vi "Hardware Config.vi"() -> ()   [LabVIEW 2022 SP3]
uses:
  Controls/Config.ctl
  Global 1.vi
panel:
  in  "Signal list":bool
  out "Config":T1={"AO config"=[], "AI config"=[], "DI config"=[], "DO config"=[], "TC config"=[{"Channel_Name"="", "Channel_Number"="", "Pre_Scale_min"=0.0, "Pre_Scale_max"=0.0, "units"=4, " type"=7}], "ACC config"=[], "SG config"=[], "Strain Gauge Settings"={"poisson ratio"=0.3, "nominal gage resistance"=120.0, "gage factor"=2.08}, "bridge information"={"strain configuration"=10271, "lead wire resistance"=1.7, "initial bridge voltage"=0.0, "voltage excitation source"=10200, "voltage excitation value"=3.3}, "Sample Rate"={"AI Sample Rate"=0.0, "AO Sample Rate"=0.0, "DI Sample Rate"=0.0, "TC Sample Rate"=0.0, "DO Sample Rate"=0.0, "SG Sample Rate"=0.0, "ACC Sample Rate"=0.0}} {"bridge information"."voltage excitation source" items=["Internal"=10200, "External"=10167, "None"=10230]; "bridge information"."voltage excitation value" format="%0.2f"; "bridge information"."lead wire resistance" format="%0.2f"; "bridge information"."strain configuration" items=["Full Bridge I"=10183, "Full Bridge II"=10184, "Full Bridge III"=10185, "Half Bridge I"=10188, "Half Bridge II"=10189, "Quarter Bridge I"=10271, "Quarter Bridge II"=10272]; "ACC config"."Terminal configuration" items=["default"=-1, "RSE"=10083, "NRSE"=10078, "Differential"=10106, "Pseudodifferential"=12529]; "ACC config"."Sensitivity units" items=["mVolts/g"=12509, "Volts/g"=12510]; "TC config"."type" items=["J"=10072, "K"=10073, "N"=10077, "R"=10082, "S"=10085, "T"=10086, "B"=10047, "E"=10055]; "TC config"."units" items=["Deg C", "Deg F", "Kelvins", "Deg R", "From Custom Scale"]}
  in  "Cancel":bool
  in  "Load Configuration":bool
  in  "New configuration":bool
  in  "Save Config":bool
  in  "Tab Control":T2(tab)
  in  "DO Sample Rate":dbl format="%#_g Hz"
  in  "DO config":T3(array[cluster])=[{"Channel_Name"="", "Channel_Number"="", "Default_Value"=FALSE, "Units"=FALSE}]
  in  "DI Sample Rate":dbl format="%#_g Hz"
  in  "DI config":T3(array[cluster])
  in  "AO Sample Rate":dbl format="%#_g Hz"
  in  "AO config":T4(array[cluster])
  in  "AI Sample Rate":dbl format="%#_g Hz"
  in  "AI config":T5(array[cluster])
  in  "TC Sample Rate":dbl format="%#_g Hz"
  in  "TC config":T6(array[cluster]) {"thermocouple type" items=["J", "K", "N", "R", "S", "T", "B", "E"]; "units" items=["Deg C", "Deg F", "Kelvins", "Deg R", "From Custom Scale"]}
  in  "ACC Sample Rate":dbl format="%#_g Hz"
  in  "ACC config":T7(array[cluster]) {"Sensitivity units" items=["mVolts/g"=12509, "Volts/g"=12510]; "Terminal configuration" items=["default"=-1, "RSE"=10083, "NRSE"=10078, "Differential"=10106, "Pseudodifferential"=12529]}
  in  "SG Sample Rate":dbl format="%#_g Hz"
  in  "SG config":T8(array[cluster])
  in  "SG Settings":T9={"gage factor"=2.08, "nominal gage \nresistance"=120.0, "poisson ratio"=0.3}
  in  "Bridge Settings":T10={"strain configuration"=10271, "lead wire resistance"=1.7, "initial bridge voltage"=0.0, "voltage excitation source"=10200, "voltage excitation value"=3.3} {"strain configuration" items=["Full Bridge I"=10183, "Full Bridge II"=10184, "Full Bridge III"=10185, "Half Bridge I"=10188, "Half Bridge II"=10189, "Quarter Bridge I"=10271, "Quarter Bridge II"=10272]; "voltage excitation source" items=["Internal"=10200, "External"=10167, "None"=10230]}
  # "DO_Channel_Name"
  # "DO_Channel_Number"
  # "Default Value"
  # "Invert?"
  # "DI_Channel_Name"
  # "DI_Channel_Number"
  # "Default Value"
  # "Invert?"
  # "AO_Channel_Name"
  # "AO_Channel_Number"
  # "Default Value"
  # "Units"
  # "AI_Channel_Name"
  # "AI_Channel_Number"
  # "Pre_Scale_min"
  # "Pre_Scale_max"
  # "Scale_min"
  # "Scale_max"
  # "Units"
  # "TC_Channel_Name"
  # "TC_Channel_Number"
  # "Max_Value"
  # "Units"
  # "Type"
  # "Min_Value"
  # "ACC_Channel_Name"
  # "ACC_Channel_Number"
  # "Min_Value"
  # "Max_Value"
  # "Terminal Config"
  # "Sensitivity"
  # "Sensitivity Units"
  # "SG_Channel_Name"
  # "SG_Channel_Number"
  # "Min_Value"
  # "Max_Value"
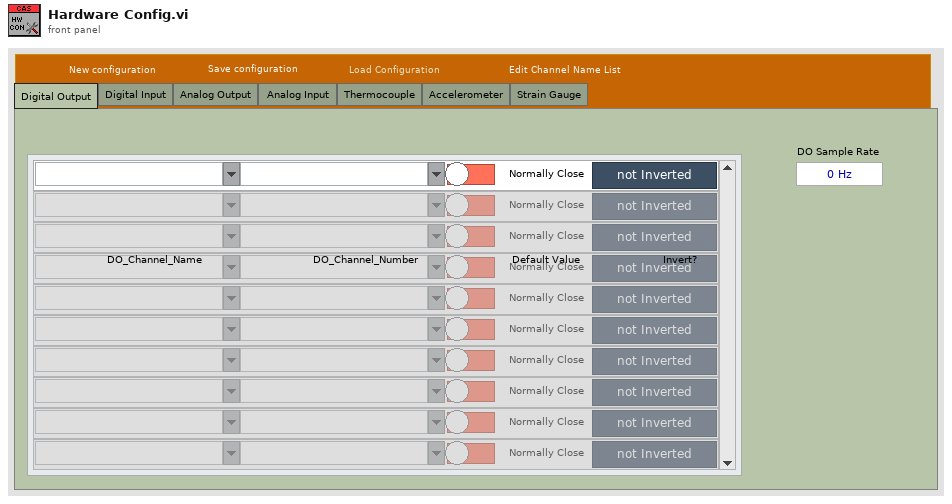
[diagram p1: front panel]
types:
  T1 = typedef "Config.ctl" = cluster{"AO config":cluster{"Channel_Name":string, "Channel_Number":string, "Default_Value":dbl, "Units":string}[], "AI config":cluster{"Channel_Name":string, "Channel_Number":string, "Pre_Scale_min":dbl, "Pre_Scale_max":dbl, "Sensor_min":dbl, "Sensor_max":dbl, "Units":string}[], "DI config":cluster{"Channel_Name":string, "Channel_Number":string, "Default_Value":bool, "DI invert?":bool}[], "DO config":cluster{"Channel_Name":string, "Channel_Number":string, "Default_Value":bool, "DO invert?":bool}[], "TC config":cluster{"Channel_Name":string, "Channel_Number":string, "Pre_Scale_min":dbl, "Pre_Scale_max":dbl, "units":i32, " type":i32}[], "ACC config":cluster{"Channel_Name":string, "Channel_Number":string, "Pre_Scale_min":dbl, "Pre_Scale_max":dbl, "Terminal configuration":i32, "Sensitivity":dbl, "Sensitivity units":i32}[], "SG config":cluster{"Channel_Name":string, "Channel_Number":string, "Pre_Scale_min":dbl, "Pre_Scale_max":dbl}[], "Strain Gauge Settings":cluster{"poisson ratio":dbl, "nominal gage resistance":dbl, "gage factor":dbl}, "bridge information":cluster{"strain configuration":i32, "lead wire resistance":dbl, "initial bridge voltage":dbl, "voltage excitation source":i32, "voltage excitation value":dbl}, "Sample Rate":cluster{"AI Sample Rate":dbl, "AO Sample Rate":dbl, "DI Sample Rate":dbl, "TC Sample Rate":dbl, "DO Sample Rate":dbl, "SG Sample Rate":dbl, "ACC Sample Rate":dbl}}
  T2 = enum32{"Digital Output", "Digital Input", "Analog Output", "Analog Input ", "Thermocouple", "Accelerometer", "Strain Gauge"}
  T3 = cluster{"Channel_Name":string, "Channel_Number":string, "Default_Value":bool, "Units":bool}[]
  T4 = cluster{"Channel_Name":string, "Channel_Number":string, "Default_Value":dbl, "Units":string}[]
  T5 = cluster{"Channel_Name":string, "Channel_Number":string, "Pre_Scale_min":dbl, "Pre_Scale_max":dbl, "Sensor_min":dbl, "Sensor_max":dbl, "Units":string}[]
  T6 = cluster{"Channel_Name":string, "Channel_Number":string, "Pre_Scale_min":dbl, "Pre_Scale_max":dbl, "units":i32, "thermocouple type":i32}[]
  T7 = cluster{"Channel_Name":string, "Channel_Number":string, "Pre_Scale_min":dbl, "Pre_Scale_max":dbl, "Terminal configuration":i32, "Sensitivity":dbl, "Sensitivity units":i32}[]
  T8 = cluster{"Channel_Name":string, "Channel_Number":string, "Pre_Scale_min":dbl, "Pre_Scale_max":dbl}[]
  T9 = cluster{"gage factor":dbl, "nominal gage \nresistance":dbl, "poisson ratio":dbl}
  T10 = cluster{"strain configuration":i32, "lead wire resistance":dbl, "initial bridge voltage":dbl, "voltage excitation source":i32, "voltage excitation value":dbl}
  T11 = cluster{"Data":T1, "path":path, "Name ref":refnum<vi>[], "Names":string[][], "Signal path":path, "SR":cluster{"AI Sample Rate":dbl, "AO Sample Rate":dbl, "DI Sample Rate":dbl, "TC Sample Rate":dbl, "DO Sample Rate":dbl, "SG Sample Rate":dbl, "ACC Sample Rate":dbl}}
  T12 = typedef "Root path.ctl" = cluster{"Data":path, "Sub VI's":path, "Source code":path}
  T13 = cluster{"AI":string[], "DI":string[], "DO":string[], "SG":string[], "AO":string[], "TC":string[], "ACC":string[]}
  T14 = cluster{"AI Channel list":tag[], "AO Channel list":tag[], "DO Channel list ":tag[], "DI Channel list":tag[]}
  T15 = cluster{"AI Sample Rate":dbl, "AO Sample Rate":dbl, "DI Sample Rate":dbl, "TC Sample Rate":dbl, "DO Sample Rate":dbl, "SG Sample Rate":dbl, "ACC Sample Rate":dbl}
  T16 = enum16{"open", "replace", "create", "open or create", "replace or create", "replace or create with confirmation"}
  T17 = enum32{"Invalid", "Standard", "Closed", "Hidden", "Minimized", "Maximized"}
  T18 = cluster{"Channel_Name":string, "Channel_Number":string, "Default_Value":bool, "DI invert?":bool}[]
  T19 = cluster{"Channel_Name":string, "Channel_Number":string, "Default_Value":bool, "DO invert?":bool}[]
  T20 = cluster{"Channel_Name":string, "Channel_Number":string, "Pre_Scale_min":dbl, "Pre_Scale_max":dbl, "units":i32, " type":i32}[]
  T21 = cluster{"poisson ratio":dbl, "nominal gage resistance":dbl, "gage factor":dbl}
  T22 = cluster{"Channel_Name":string, "Channel_Number":string}
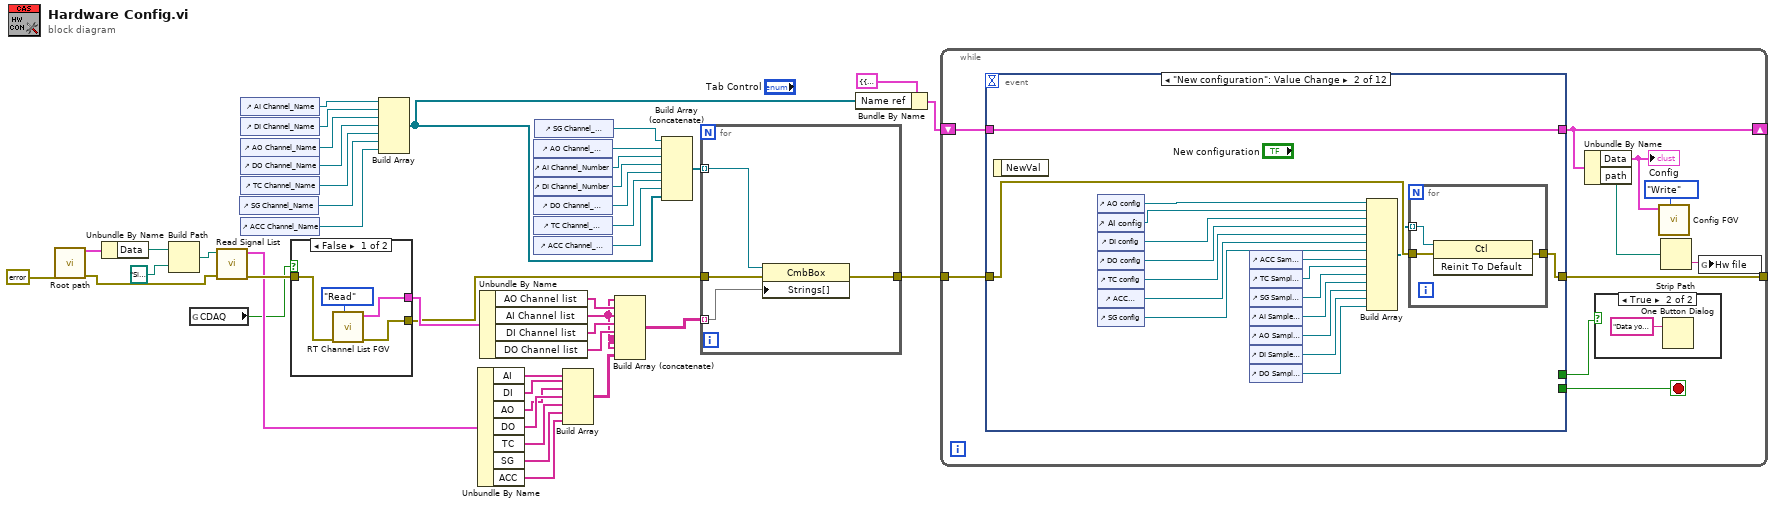
[diagram p0: block diagram]
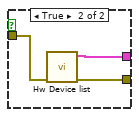
[diagram p2: hidden frame]
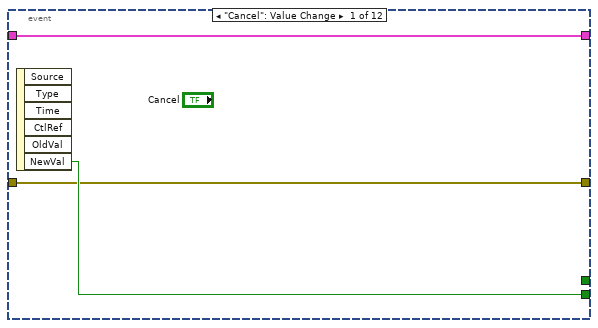
[diagram p4: hidden frame]
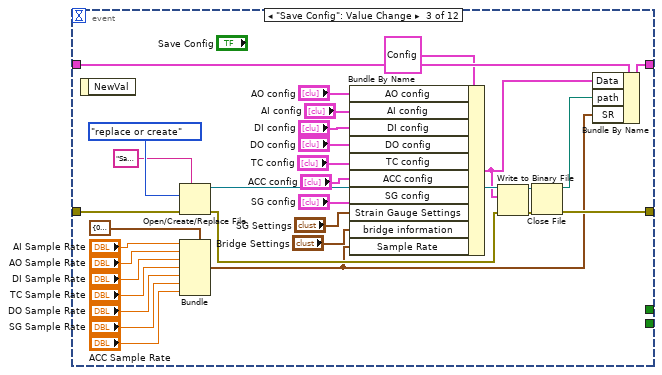
[diagram p5: hidden frame]
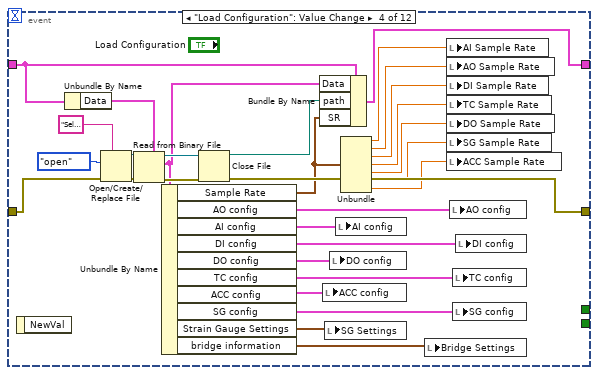
[diagram p6: hidden frame]
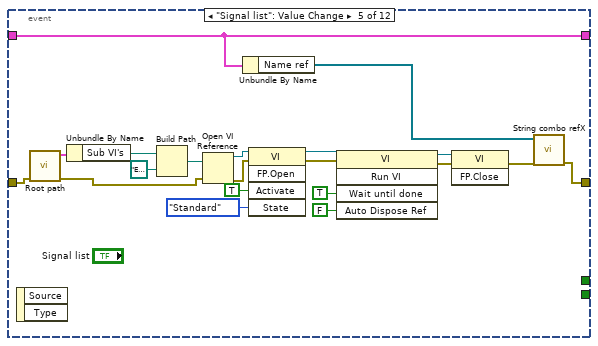
[diagram p7: hidden frame]
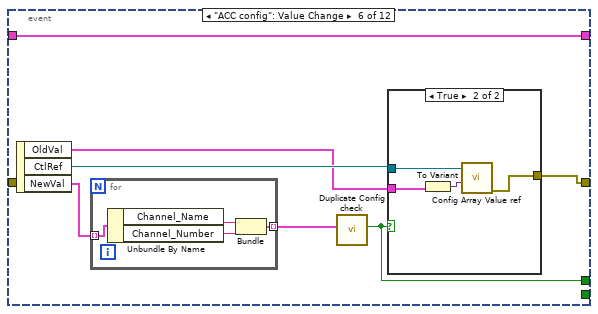
[diagram p8: hidden frame]
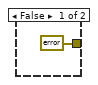
[diagram p9: hidden frame]
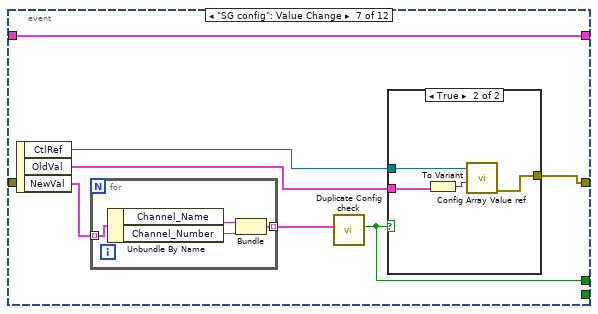
[diagram p10: hidden frame]
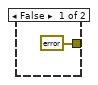
[diagram p11: hidden frame]
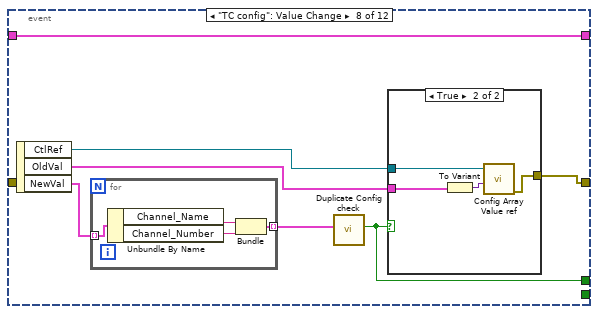
[diagram p12: hidden frame]
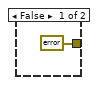
[diagram p13: hidden frame]
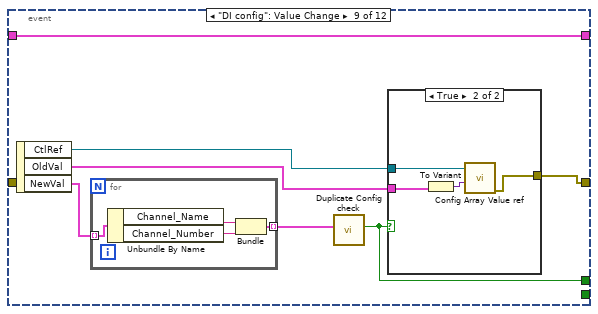
[diagram p14: hidden frame]
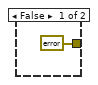
[diagram p15: hidden frame]
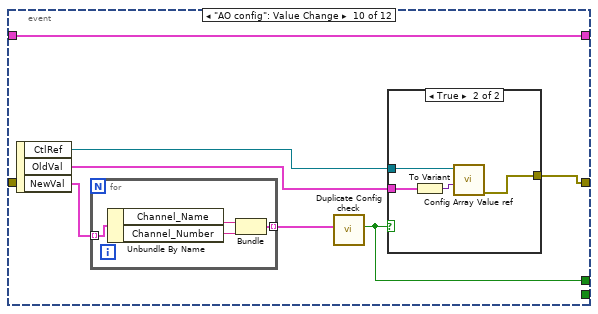
[diagram p16: hidden frame]
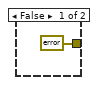
[diagram p17: hidden frame]
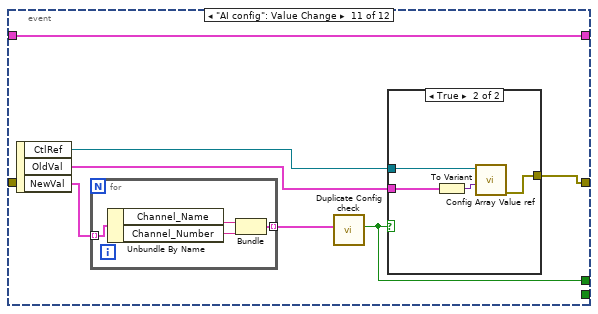
[diagram p18: hidden frame]
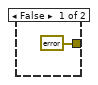
[diagram p19: hidden frame]
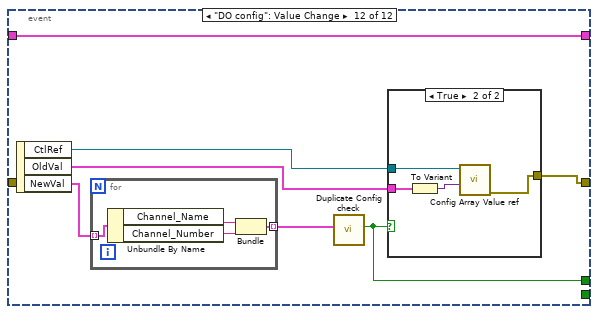
[diagram p20: hidden frame]
diagram:
  n1 = call "Root path.vi"("error in (no error)"=errorcluster {"status"=FALSE, "code"=0, "source"=""} ("error in")) -> ("error out"=w18:errorcluster, "Root Path"=w25:T12)  [unwired: 9 in]
  n2 = Unbundle By Name(w25) -> ("Data"=w24:path)
  n3 = Build Path(base path=w24, name or relative path=path "Signal list/Signal1") -> (appended path=w22:path)
  n4 = global read "Global 1.vi" "CDAQ"() -> (w1:bool)
  n5 = call "Read Signal List.vi"("error in"=w18, "file path (use dialog)"=w22) -> ("error out"=w27:errorcluster, "Names"=w17:T13)  [unwired: 8 in]
  n6 = control-ref of="SG Channel_Name"() -> (w3:refnum<vi>)
  n7 = control-ref of="AI Channel_Name"() -> (w21:refnum<vi>)
  n8 = control-ref of="DI Channel_Name"() -> (w20:refnum<vi>)
  n9 = control-ref of="AO Channel_Name"() -> (w5:refnum<vi>)
  n10 = control-ref of="DO Channel_Name"() -> (w4:refnum<vi>)
  n11 = control-ref of="TC Channel_Name"() -> (w19:refnum<vi>)
  n12 = control-ref of="ACC Channel_Name"() -> (w2:refnum<vi>)
  n13 = case shown="False" w1 {
    tunnel: [w46 w50] -> w35
    tunnel: [w45 w49] -> w34
    tunnel: w27 -> [w44 w48]
    frame False {
      n14 = call "RT Channel List FGV.vi"("Enum"=enum16{"Read", "Write"}."Read", "error in (no error)"=w44) -> ("error out"=w45:errorcluster, "Channel List"=w46:T14)  [unwired: 8 in]
    }
    frame True {
      n15 = call "Hw Device list.vi"("error in (no error)"=w48) -> ("error out"=w49:errorcluster, "Channel List"=w50:T14)  [unwired: 9 in]
    }
  }
  n16 = Build Array(w21, w20, w5, w4, w19, w3, w2) -> (w6:refnum<vi>[])
  n17 = Unbundle By Name(w17) -> ("AI"=w16:string[], "DI"=w15:string[], "AO"=w10:string[], "DO"=w14:string[], "TC"=w13:string[], "SG"=w12:string[], "ACC"=w11:string[])
  n18 = Unbundle By Name(w35) -> ("AO Channel list"=w29:tag[], "AI Channel list"=w28:tag[], "DI Channel list"=w38:tag[], "DO Channel list"=w37:tag[])
  n19 = control-ref of="AO Channel_Number"() -> (w43:refnum<vi>)
  n20 = control-ref of="AI Channel_Number"() -> (w42:refnum<vi>)
  n21 = control-ref of="DI Channel_Number"() -> (w41:refnum<vi>)
  n22 = control-ref of="DO Channel_Number"() -> (w40:refnum<vi>)
  n23 = control-ref of="TC Channel_Number"() -> (w32:refnum<vi>)
  n24 = control-ref of="ACC Channel_Number"() -> (w31:refnum<vi>)
  n25 = control-ref of="SG Channel_Number"() -> (w30:refnum<vi>)
  n26 = Build Array(w16, w15, w10, w14, w13, w12, w11) -> (w9:string[][])
  n27 = Build Array (concatenate)(w28, w29, w28, w38, w37, w28, w28, w9) -> (w36:string[][])
  n28 = Build Array (concatenate)(w30, w43, w42, w41, w40, w32, w31, w6) -> (w39:refnum<vi>[])
  n29 = for {
    tunnel: w39 -> [w54] mode=indexing
    tunnel: w36 -> [w51] mode=indexing
    tunnel: [w53] -> w33
    tunnel: w34 -> [w52]
    n30 = property class="CmbBox"(reference=w54, error in=w52, "Strings[]"=w51) -> (error out=w53:errorcluster)  [unwired: 1 out]
  }
  n31 = Bundle By Name(cluster=T11 {"Data"={"AO config"=[], "AI config"=[], "DI config"=[], "DO config"=[], "TC config"=[{"Channel_Name"="", "Channel_Number"="", "Pre_Scale_min"=0.0, "Pre_Scale_max"=0.0, "units"=4, " type"=7}], "ACC config"=[], "SG config"=[], "Strain Gauge Settings"={"poisson ratio"=0.3, "nominal gage resistance"=120.0, "gage factor"=2.08}, "bridge information"={"strain configuration"=10271, "lead wire resistance"=1.7, "initial bridge voltage"=0.0, "voltage excitation source"=10200, "voltage excitation value"=3.3}, "Sample Rate"={"AI Sample Rate"=0.0, "AO Sample Rate"=0.0, "DI Sample Rate"=0.0, "TC Sample Rate"=0.0, "DO Sample Rate"=0.0, "SG Sample Rate"=0.0, "ACC Sample Rate"=0.0}}, "path"=path "", "Name ref"=[], "Names"=[], "Signal path"=path "", "SR"={"AI Sample Rate"=0.0, "AO Sample Rate"=0.0, "DI Sample Rate"=0.0, "TC Sample Rate"=0.0, "DO Sample Rate"=0.0, "SG Sample Rate"=0.0, "ACC Sample Rate"=0.0}}, "Name ref"=w6) -> (w8:T11)
  n32 = while {
    shift-right: [w60] -> _
    shift-left: w8 -> [w61]
    tunnel: w33 -> [w63]
    tunnel: [w62] -> _
    stop <- w64 stop-if-true
    n33 = event shown="[1] \"New configuration\": Value Change" {
      selector: _ -> [_ _ _ _ _ _ _ _ _ _ _ _]
      dyn-events: _ -> [_ _ _ _ _ _ _ _ _ _ _ _]
      timeout: _ -> [_ _ _ _ _ _ _ _ _ _ _ _]
      tunnel: [w67 _ _ _ _ _ _ _ _ _ _ _] -> w64
      tunnel: w63 -> [w66 w86 w120 w150 w170 _ _ _ _ _ _ _]
      tunnel: [w66 w85 w115 w146 w151 w172 w190 w206 w222 w238 w254 w270] -> w62
      tunnel: w61 -> [w68 w84 w118 w140 w154 w177 w193 w209 w225 w241 w257 w273]
      tunnel: [w68 w84 w107 w141 w154 w177 w193 w209 w225 w241 w257 w273] -> w60
      tunnel: [_ _ _ _ _ w171 w187 w203 w219 w235 w251 w267] -> w55
      event "Cancel": Value Change {
        n34 = event-data() -> ("NewVal"=w67:bool)  [unwired: 1 in, 5 out]
      }
      event "New configuration": Value Change {
        n35 = event-data() -> ()  [unwired: 1 in, 1 out]
        n36 = control-ref of="AO config"() -> (w79:refnum<vi>)
        n37 = control-ref of="AI config"() -> (w80:refnum<vi>)
        n38 = control-ref of="DI config"() -> (w81:refnum<vi>)
        n39 = control-ref of="DO config"() -> (w82:refnum<vi>)
        n40 = control-ref of="TC config"() -> (w78:refnum<vi>)
        n41 = control-ref of="ACC config"() -> (w77:refnum<vi>)
        n42 = control-ref of="SG config"() -> (w76:refnum<vi>)
        n43 = control-ref of="ACC Sample Rate"() -> (w75:refnum<vi>)
        n44 = control-ref of="TC Sample Rate"() -> (w74:refnum<vi>)
        n45 = control-ref of="SG Sample Rate"() -> (w73:refnum<vi>)
        n46 = control-ref of="AI Sample Rate"() -> (w72:refnum<vi>)
        n47 = control-ref of="AO Sample Rate"() -> (w71:refnum<vi>)
        n48 = control-ref of="DI Sample Rate"() -> (w70:refnum<vi>)
        n49 = control-ref of="DO Sample Rate"() -> (w69:refnum<vi>)
        n50 = Build Array(w79, w80, w81, w82, w78, w77, w76, w75, w74, w73, w72, w71, w70, w69) -> (w83:refnum<vi>[])
        n51 = for {
          tunnel: w83 -> [w89] mode=indexing
          tunnel: w86 -> [w88]
          tunnel: [w87] -> w85
          n52 = invoke class="Ctl" method="Reinit To Default"(reference=w89, error in=w88) -> (error out=w87:errorcluster)  [unwired: 1 in, 2 out]
        }
      }
      event "Save Config": Value Change {
        n53 = event-data() -> ()  [unwired: 1 in, 1 out]
        n54 = Open/Create/Replace File(error in=w120, prompt="Save Changes", operation (0:open)=T16."replace or create") -> (refnum out=w114:refnum<file>, error out=w119:errorcluster)  [unwired: 3 in, 1 out]
        n55 = Bundle(cluster=T15 {"AI Sample Rate"=0.0, "AO Sample Rate"=0.0, "DI Sample Rate"=0.0, "TC Sample Rate"=0.0, "DO Sample Rate"=0.0, "SG Sample Rate"=0.0, "ACC Sample Rate"=0.0} ("Sample Rate"), "AI Sample Rate"="AI Sample Rate", "AO Sample Rate"="AO Sample Rate", "DI Sample Rate"="DI Sample Rate", "TC Sample Rate"="TC Sample Rate", "DO Sample Rate"="DO Sample Rate", "SG Sample Rate"="SG Sample Rate", "ACC Sample Rate"="ACC Sample Rate") -> (w90:T15)
        n56 = Bundle By Name(cluster=T1 {"AO config"=[], "AI config"=[], "DI config"=[], "DO config"=[], "TC config"=[{"Channel_Name"="", "Channel_Number"="", "Pre_Scale_min"=0.0, "Pre_Scale_max"=0.0, "units"=4, " type"=7}], "ACC config"=[], "SG config"=[], "Strain Gauge Settings"={"poisson ratio"=0.3, "nominal gage resistance"=120.0, "gage factor"=2.08}, "bridge information"={"strain configuration"=10271, "lead wire resistance"=1.7, "initial bridge voltage"=0.0, "voltage excitation source"=10200, "voltage excitation value"=3.3}, "Sample Rate"={"AI Sample Rate"=0.0, "AO Sample Rate"=0.0, "DI Sample Rate"=0.0, "TC Sample Rate"=0.0, "DO Sample Rate"=0.0, "SG Sample Rate"=0.0, "ACC Sample Rate"=0.0}} ("Data"), "AO config"="AO config", "AI config"="AI config", "DI config"="DI config", "DO config"="DO config", "TC config"="TC config", "ACC config"="ACC config", "SG config"="SG config", "Strain Gauge Settings"="SG Settings", "bridge information"="Bridge Settings", "Sample Rate"=w90) -> (w105:T1)
        n57 = Write to Binary File(file (use dialog)=w114, data=w105, error in=w119) -> (refnum out=w117:refnum<file>, error out=w116:errorcluster)  [unwired: 3 in, 1 out]
        n58 = Close File(refnum=w117, error in=w116) -> (path=w101:path, error out=w115:errorcluster)
        n59 = Bundle By Name(cluster=w118, "Data"=w105, "path"=w101, "SR"=w90) -> (w107:T11)
      }
      event "Load Configuration": Value Change {
        n60 = event-data() -> ()  [unwired: 1 in, 1 out]
        n61 = Unbundle By Name(w140) -> ("Data"=w142:T1)
        n62 = Open/Create/Replace File(error in=w150, prompt="Select file to load", operation (0:open)=T16."open") -> (refnum out=w145:refnum<file>, error out=w149:errorcluster)  [unwired: 3 in, 1 out]
        n63 = Read from Binary File(5:w142, 8:w149, 11:w145) -> (0:w147:errorcluster, 2:w139:T1, 3:w148:refnum<file>)  [unwired: 3 in, 1 out]
        n64 = Unbundle By Name(w139) -> ("Sample Rate"=w128:T15, "AO config"=w138:T4, "AI config"=w137:T5, "DI config"=w136:T18, "DO config"=w135:T19, "TC config"=w134:T20, "ACC config"=w133:T7, "SG config"=w132:T8, "Strain Gauge Settings"=w130:T21, "bridge information"=w129:T10)
        n65 = Close File(refnum=w148, error in=w147) -> (path=w131:path, error out=w146:errorcluster)
        n66 = Bundle By Name(cluster=w140, "Data"=w139, "path"=w131, "SR"=w128) -> (w141:T11)
        n67 = local write "ACC config"(w133) -> ()
        n68 = local write "SG Settings"(w130) -> ()
        n69 = local write "DO config"(w135) -> ()
        n70 = local write "AI config"(w137) -> ()
        n71 = Unbundle(w128) -> ("AI Sample Rate"=w127:dbl, "AO Sample Rate"=w126:dbl, "DI Sample Rate"=w125:dbl, "TC Sample Rate"=w124:dbl, "DO Sample Rate"=w123:dbl, "SG Sample Rate"=w122:dbl, "ACC Sample Rate"=w121:dbl)
        n72 = local write "Bridge Settings"(w129) -> ()
        n73 = local write "AI Sample Rate"(w127) -> ()
        n74 = local write "AO Sample Rate"(w126) -> ()
        n75 = local write "DI Sample Rate"(w125) -> ()
        n76 = local write "TC Sample Rate"(w124) -> ()
        n77 = local write "DO Sample Rate"(w123) -> ()
        n78 = local write "SG Sample Rate"(w122) -> ()
        n79 = local write "ACC Sample Rate"(w121) -> ()
        n80 = local write "AO config"(w138) -> ()
        n81 = local write "TC config"(w134) -> ()
        n82 = local write "SG config"(w132) -> ()
        n83 = local write "DI config"(w136) -> ()
      }
      event "Signal list": Value Change {
        n84 = event-data() -> ()  [unwired: 1 in, 2 out]
        n85 = call "Root path.vi"("error in (no error)"=w170) -> ("error out"=w165:errorcluster, "Root Path"=w169:T12)  [unwired: 9 in]
        n86 = Unbundle By Name(w169) -> ("Sub VI's"=w168:path)
        n87 = Build Path(base path=w168, name or relative path=path "Edit Channel Name list.vi") -> (appended path=w166:path)
        n88 = Open VI Reference(vi path=w166, error in (no error)=w165) -> (vi reference=w156:refnum<vi>, error out=w155:errorcluster)  [unwired: 4 in]
        n89 = Unbundle By Name(w154) -> ("Name ref"=w153:refnum<vi>[])
        n90 = invoke class="VI" method="FP.Open"(reference=w156, error in=w155, "Activate"=TRUE ("Activate?"), "State"=T17."Standard") -> (reference out=w164:refnum<vi>, error out=w163:errorcluster)  [unwired: 1 in, 3 out]
        n91 = invoke class="VI" method="Run VI"(reference=w164, error in=w163, "Wait until done"=TRUE ("Wait Until Done"), "Auto Dispose Ref"=FALSE ("Auto Dispose Reference")) -> (reference out=w162:refnum<vi>, error out=w161:errorcluster)  [unwired: 1 in, 3 out]
        n92 = invoke class="VI" method="FP.Close"(reference=w162, error in=w161) -> (error out=w152:errorcluster)  [unwired: 1 in, 2 out]
        n93 = call "String combo refX.vi"("error out"=w152, "Ctrl ref"=w153) -> ("error out 2"=w151:errorcluster)  [unwired: 9 in]
      }
      event "ACC config": Value Change {
        n94 = event-data() -> ("OldVal"=w173:T7, "CtlRef"=w174:refnum<vi>, "NewVal"=w176:T7)  [unwired: 1 in]
        n95 = for {
          tunnel: w176 -> [w181] mode=indexing
          tunnel: [w178] -> w175 mode=indexing
          n96 = Unbundle By Name(w181) -> ("Channel_Name"=w179:string, "Channel_Number"=w180:string)
          n97 = Bundle("Channel_Name"=w179, "Channel_Number"=w180) -> (w178:T22)  [unwired: 1 in]
        }
        n98 = call "Duplicate Config check.vi"("Data in"=w175) -> ("Channel list indication"=w171:bool)  [unwired: 10 in]
        n99 = case shown="True" w171 {
          tunnel: w174 -> [_ w185]
          tunnel: w173 -> [_ w184]
          tunnel: [errorcluster {"status"=FALSE, "code"=0, "source"=""} ("error out") w183] -> w172
          frame False {
          }
          frame True {
            n100 = To Variant(anything=w184) -> (Variant=w186:variant)
            n101 = call "Config Array Value ref.vi"("Value"=w186, "Array in"=w185) -> ("error out"=w183:errorcluster)  [unwired: 9 in]
          }
        }
      }
      event "SG config": Value Change {
        n102 = event-data() -> ("CtlRef"=w189:refnum<vi>, "OldVal"=w188:T8, "NewVal"=w192:T8)  [unwired: 1 in]
        n103 = for {
          tunnel: w192 -> [w197] mode=indexing
          tunnel: [w194] -> w191 mode=indexing
          n104 = Unbundle By Name(w197) -> ("Channel_Name"=w195:string, "Channel_Number"=w196:string)
          n105 = Bundle("Channel_Name"=w195, "Channel_Number"=w196) -> (w194:T22)  [unwired: 1 in]
        }
        n106 = call "Duplicate Config check.vi"("Data in"=w191) -> ("Channel list indication"=w187:bool)  [unwired: 10 in]
        n107 = case shown="True" w187 {
          tunnel: w189 -> [_ w201]
          tunnel: w188 -> [_ w200]
          tunnel: [errorcluster {"status"=FALSE, "code"=0, "source"=""} ("error out") w199] -> w190
          frame False {
          }
          frame True {
            n108 = To Variant(anything=w200) -> (Variant=w202:variant)
            n109 = call "Config Array Value ref.vi"("Value"=w202, "Array in"=w201) -> ("error out"=w199:errorcluster)  [unwired: 9 in]
          }
        }
      }
      event "TC config": Value Change {
        n110 = event-data() -> ("CtlRef"=w205:refnum<vi>, "OldVal"=w204:T6, "NewVal"=w208:T6)  [unwired: 1 in]
        n111 = for {
          tunnel: w208 -> [w213] mode=indexing
          tunnel: [w210] -> w207 mode=indexing
          n112 = Unbundle By Name(w213) -> ("Channel_Name"=w211:string, "Channel_Number"=w212:string)
          n113 = Bundle("Channel_Name"=w211, "Channel_Number"=w212) -> (w210:T22)  [unwired: 1 in]
        }
        n114 = call "Duplicate Config check.vi"("Data in"=w207) -> ("Channel list indication"=w203:bool)  [unwired: 10 in]
        n115 = case shown="True" w203 {
          tunnel: w205 -> [_ w217]
          tunnel: w204 -> [_ w216]
          tunnel: [errorcluster {"status"=FALSE, "code"=0, "source"=""} ("error out") w215] -> w206
          frame False {
          }
          frame True {
            n116 = To Variant(anything=w216) -> (Variant=w218:variant)
            n117 = call "Config Array Value ref.vi"("Value"=w218, "Array in"=w217) -> ("error out"=w215:errorcluster)  [unwired: 9 in]
          }
        }
      }
      event "DI config": Value Change {
        n118 = event-data() -> ("CtlRef"=w221:refnum<vi>, "OldVal"=w220:T3, "NewVal"=w224:T3)  [unwired: 1 in]
        n119 = for {
          tunnel: w224 -> [w229] mode=indexing
          tunnel: [w226] -> w223 mode=indexing
          n120 = Unbundle By Name(w229) -> ("Channel_Name"=w227:string, "Channel_Number"=w228:string)
          n121 = Bundle("Channel_Name"=w227, "Channel_Number"=w228) -> (w226:T22)  [unwired: 1 in]
        }
        n122 = call "Duplicate Config check.vi"("Data in"=w223) -> ("Channel list indication"=w219:bool)  [unwired: 10 in]
        n123 = case shown="True" w219 {
          tunnel: w221 -> [_ w233]
          tunnel: w220 -> [_ w232]
          tunnel: [errorcluster {"status"=FALSE, "code"=0, "source"=""} ("error out") w231] -> w222
          frame False {
          }
          frame True {
            n124 = To Variant(anything=w232) -> (Variant=w234:variant)
            n125 = call "Config Array Value ref.vi"("Value"=w234, "Array in"=w233) -> ("error out"=w231:errorcluster)  [unwired: 9 in]
          }
        }
      }
      event "AO config": Value Change {
        n126 = event-data() -> ("CtlRef"=w237:refnum<vi>, "OldVal"=w236:T4, "NewVal"=w240:T4)  [unwired: 1 in]
        n127 = for {
          tunnel: w240 -> [w245] mode=indexing
          tunnel: [w242] -> w239 mode=indexing
          n128 = Unbundle By Name(w245) -> ("Channel_Name"=w243:string, "Channel_Number"=w244:string)
          n129 = Bundle("Channel_Name"=w243, "Channel_Number"=w244) -> (w242:T22)  [unwired: 1 in]
        }
        n130 = call "Duplicate Config check.vi"("Data in"=w239) -> ("Channel list indication"=w235:bool)  [unwired: 10 in]
        n131 = case shown="True" w235 {
          tunnel: w237 -> [_ w250]
          tunnel: w236 -> [_ w248]
          tunnel: [errorcluster {"status"=FALSE, "code"=0, "source"=""} ("error out") w249] -> w238
          frame False {
          }
          frame True {
            n132 = To Variant(anything=w248) -> (Variant=w247:variant)
            n133 = call "Config Array Value ref.vi"("Value"=w247, "Array in"=w250) -> ("error out"=w249:errorcluster)  [unwired: 9 in]
          }
        }
      }
      event "AI config": Value Change {
        n134 = event-data() -> ("CtlRef"=w253:refnum<vi>, "OldVal"=w252:T5, "NewVal"=w256:T5)  [unwired: 1 in]
        n135 = for {
          tunnel: w256 -> [w261] mode=indexing
          tunnel: [w258] -> w255 mode=indexing
          n136 = Unbundle By Name(w261) -> ("Channel_Name"=w259:string, "Channel_Number"=w260:string)
          n137 = Bundle("Channel_Name"=w259, "Channel_Number"=w260) -> (w258:T22)  [unwired: 1 in]
        }
        n138 = call "Duplicate Config check.vi"("Data in"=w255) -> ("Channel list indication"=w251:bool)  [unwired: 10 in]
        n139 = case shown="True" w251 {
          tunnel: w253 -> [_ w265]
          tunnel: w252 -> [_ w264]
          tunnel: [errorcluster {"status"=FALSE, "code"=0, "source"=""} ("error out") w263] -> w254
          frame False {
          }
          frame True {
            n140 = To Variant(anything=w264) -> (Variant=w266:variant)
            n141 = call "Config Array Value ref.vi"("Value"=w266, "Array in"=w265) -> ("error out"=w263:errorcluster)  [unwired: 9 in]
          }
        }
      }
      event "DO config": Value Change {
        n142 = event-data() -> ("CtlRef"=w269:refnum<vi>, "OldVal"=w268:T3, "NewVal"=w272:T3)  [unwired: 1 in]
        n143 = for {
          tunnel: w272 -> [w277] mode=indexing
          tunnel: [w274] -> w271 mode=indexing
          n144 = Unbundle By Name(w277) -> ("Channel_Name"=w275:string, "Channel_Number"=w276:string)
          n145 = Bundle("Channel_Name"=w275, "Channel_Number"=w276) -> (w274:T22)  [unwired: 1 in]
        }
        n146 = call "Duplicate Config check.vi"("Data in"=w271) -> ("Channel list indication"=w267:bool)  [unwired: 10 in]
        n147 = case shown="True" w267 {
          tunnel: w269 -> [_ w282]
          tunnel: w268 -> [_ w280]
          tunnel: [errorcluster {"status"=FALSE, "code"=0, "source"=""} ("error out") w281] -> w270
          frame False {
          }
          frame True {
            n148 = To Variant(anything=w280) -> (Variant=w279:variant)
            n149 = call "Config Array Value ref.vi"("Value"=w279, "Array in"=w282) -> ("error out"=w281:errorcluster)  [unwired: 9 in]
          }
        }
      }
    }
    n150 = Unbundle By Name(w60) -> ("Data"=w59:T1, "path"=w56:path)
    "Config" <- w59
    n151 = case shown="True" w55 {
      frame False {
      }
      frame True {
        n152 = One Button Dialog ("Warning")(message="Data you Entered is already Exist!") -> ()  [unwired: 1 in, 1 out]
      }
    }
    n153 = call "Config FGV.vi"("Enum"=enum16{"Read", "Write"}."Write", "Data 2"=w59) -> ()  [unwired: 8 in, 2 out]
    n154 = Strip Path(path=w56) -> (name=w57:string)  [unwired: 1 out]
    n155 = global write "Global 1.vi" "Hw file"(w57) -> ()
  }
